vi "Get Attribute - I32.vi"(8 "error in (no error)":errorcluster, 9 "Default Value (0)":i32, 10 "Key":string, 11 "YAML Parser in":refnum<class "YAML Parser.lvclass">) -> (0 "error out":errorcluster, 1 "Is Null?":bool, 2 "Value":i32, 3 "YAML Parser out":refnum<class "YAML Parser.lvclass">)   [LabVIEW 2015, in "YAML Parser.lvclass"]
uses:
  YAML Parser.lvclass
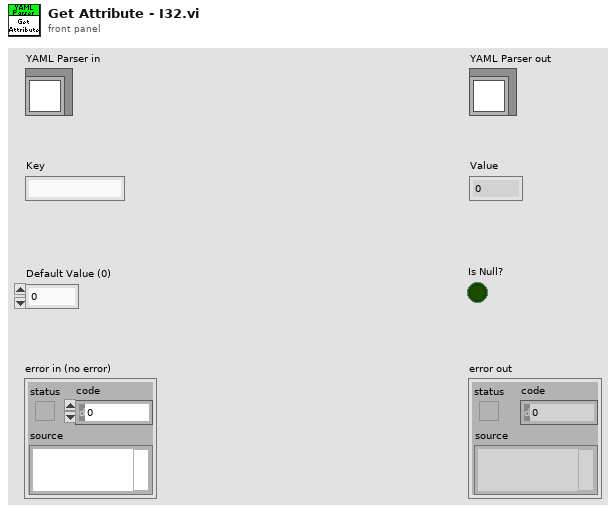
[diagram p1: front panel]
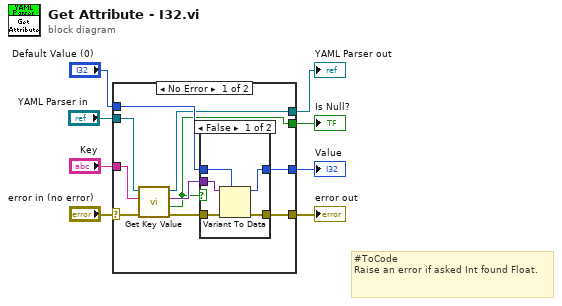
[diagram p0: block diagram]
diagram:
  # "#ToCode\nRaise an error if asked Int found Float."
  n1 = case shown="No Error" "error in (no error)" {
    selector: "error in (no error)" -> [w16 w27]
    tunnel: [w18 w27] -> w7
    tunnel: [w13 w26] -> w5
    tunnel: "YAML Parser in" -> [w14 w26]
    tunnel: "Default Value (0)" -> [w17 _]
    tunnel: "Key" -> [w11 _]
    tunnel: [w10 _] -> w2
    tunnel: [w9 _] -> w1
    frame No Error {
      n2 = call "Get Key Value.vi"("error in (no error)"=w16, "Key"=w11, "YAML Parser in"=w14) -> ("error out"=w15:errorcluster, "Is Null?"=w10:bool, "Key Value"=w12:variant, "YAML Parser out"=w13:refnum<class "YAML Parser.lvclass">)  [unwired: 5 in]
      n3 = case shown="False" w10 {
        tunnel: [w23 w25] -> w18
        tunnel: w17 -> [w22 w24]
        tunnel: w15 -> [w21 w25]
        tunnel: w12 -> [w20 _]
        tunnel: [w19 w24] -> w9
        frame False {
          n4 = Variant To Data(error in=w21, type=w22, Variant=w20) -> (data=w19:i32, error out=w23:errorcluster)
        }
        frame True {
        }
      }
    }
    frame Error {
    }
  }
  "error out" <- w7
  "YAML Parser out" <- w5
  "Value" <- w1
  "Is Null?" <- w2
